vi "KepcoDCPwr Configure Output State.vi"(0 "VISA Session":refnum<visa-resource-name>, 5 "Model In":string, 7 "channel name (\"\")":string="\"\"", 9 "Power Supply Mode":bool, 11 "error in (no error)":errorcluster {"code" format="%.0x"}) -> (4 "VISA Session Out":refnum<visa-resource-name>, 6 "Model Out":string, 8 "channel name out (\"\")":string="\"\"" caption="channel name Out (\"\")", 15 "error out":errorcluster {"code" format="%.0x"})   [LabVIEW 2013]
doc: "This VI Sets the Biolar Power Supply to operate in Voltage or current Mode\n\nMode input T=Voltage, False = Current mode of operation"
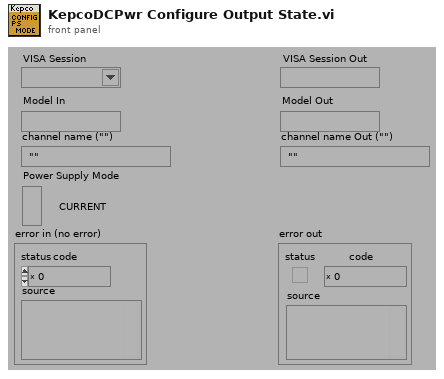
[diagram p1: front panel]
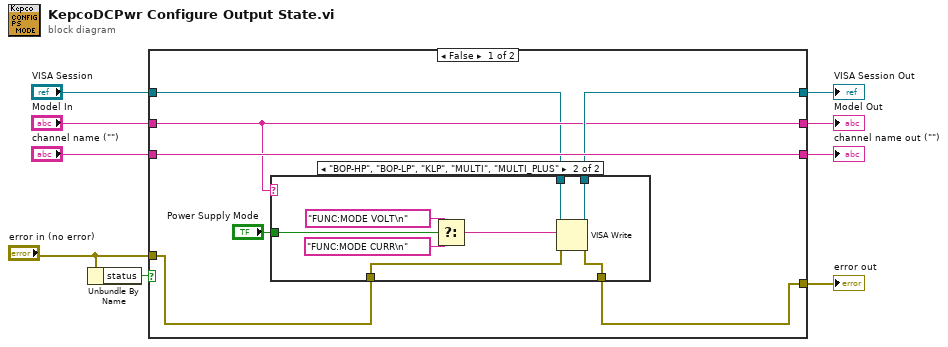
[diagram p0: block diagram]
diagram:
  n1 = Unbundle By Name("error in (no error)") -> ("status"=w8:bool)
  n2 = case shown="False" w8 {
    tunnel: [w12 w30] -> w9
    tunnel: "error in (no error)" -> [w14 w30]
    tunnel: [w15 w29] -> w3
    tunnel: "VISA Session" -> [w11 w29]
    tunnel: [w13 w28] -> w2
    tunnel: "Model In" -> [w13 w28]
    tunnel: [w16 w27] -> w1
    tunnel: "channel name (\"\")" -> [w16 w27]
    frame False {
      n3 = case shown="\"BOP-HP\", \"BOP-LP\", \"KLP\", \"MULTI\", \"MULTI_PLUS\"" w13 {
        tunnel: w14 -> [w18 w26]
        tunnel: [w18 w23] -> w12
        tunnel: [w17 w24] -> w15
        tunnel: w11 -> [w17 w25]
        tunnel: "Power Supply Mode" -> [_ w19]
        frame "", "STANDARD", Default {
        }
        frame "BOP-HP", "BOP-LP", "KLP", "MULTI", "MULTI_PLUS" {
          n4 = Select(t="FUNC:MODE VOLT\n", s=w19, f="FUNC:MODE CURR\n") -> (s? t:f=w20:string)
          n5 = VISA Write(VISA resource name=w25, write buffer=w20, error in (no error)=w26) -> (VISA resource name out=w24:refnum<visa-resource-name>, error out=w23:errorcluster)  [unwired: 1 out]
        }
      }
    }
    frame True {
    }
  }
  "error out" <- w9
  "channel name out (\"\")" <- w1
  "Model Out" <- w2
  "VISA Session Out" <- w3
